vi "UTIL Number of Samples.vi"(8 "Error In":errorcluster, 11 "Task In":refnum<k21>) -> (0 "Error Out":errorcluster, 1 "Samples/Chan":i32, 3 "Task Out":refnum<k21>)   [LabVIEW 2017]
doc: "The VI returns the number of Samples/Channel for a pre-defined Task.\n\nInputs:\n Task In DAQmx Task, already defined\n Error In\nOutputs:\n Task Out Passthrough\n Samples/Chan I32, from Task Timing Property\n Error Out"
uses:
  <resource>/objmgr/daqmx.rc
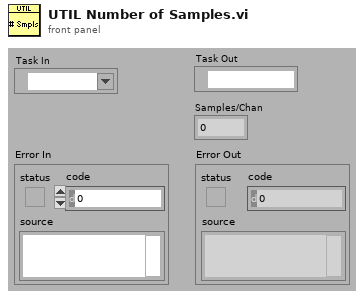
[diagram p1: front panel]
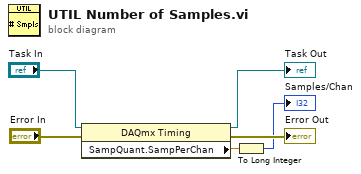
[diagram p0: block diagram]
diagram:
  n1 = property class="DAQmx Timing"(reference="Task In", error in="Error In") -> (reference out=→"Task Out":refnum<k21>, error out=→"Error Out":errorcluster, "SampQuant.SampPerChan"=w2:dbl)
  n2 = To Long Integer(number=w2) -> (32bit integer=→"Samples/Chan":i32)
